vi "실습 1-1.vi"() -> ()   [LabVIEW 2014]
panel:
  out "웨이브폼 차트":dbl(graph)
  in  "정지":bool
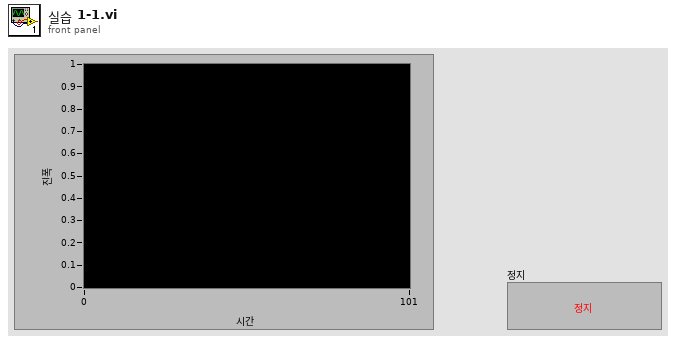
[diagram p1: front panel]
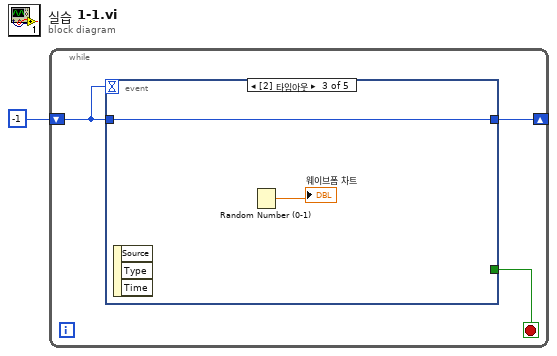
[diagram p0: block diagram]
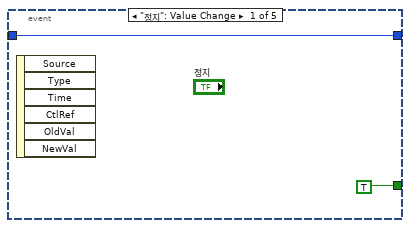
[diagram p2: hidden frame]
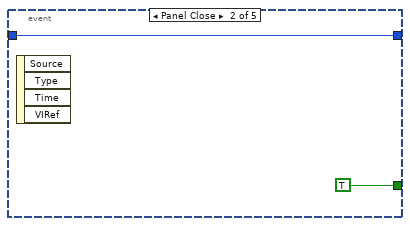
[diagram p3: hidden frame]
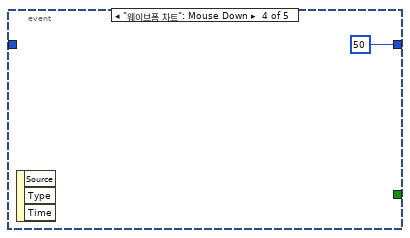
[diagram p4: hidden frame]
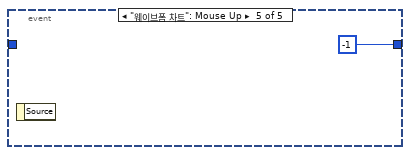
[diagram p5: hidden frame]
diagram:
  n1 = while {
    shift-right: [w3] -> _
    shift-left: -1 -> [w2]
    stop <- w4 stop-if-true
    n2 = event shown="[2] 타임아웃" {
      selector: _ -> [_ _ _ _ _]
      dyn-events: _ -> [_ _ _ _ _]
      timeout: w2 -> [_ _ _ _ _]
      tunnel: [TRUE TRUE _ _ _] -> w4
      tunnel: w2 -> [w6 w8 w10 _ _]
      tunnel: [w6 w8 w10 50 -1] -> w3
      event "정지": Value Change {
        n3 = event-data() -> ()  [unwired: 1 in, 6 out]
      }
      event Panel Close {
        n4 = event-data() -> ()  [unwired: 1 in, 4 out]
      }
      event Timeout {
        n5 = event-data() -> ()  [unwired: 1 in, 3 out]
        n6 = Random Number (0-1)() -> (number: 0 to 1=→"웨이브폼 차트":dbl)
      }
      event "웨이브폼 차트": Mouse Down {
        n7 = event-data() -> ()  [unwired: 1 in, 3 out]
      }
      event "웨이브폼 차트": Mouse Up {
        n8 = event-data() -> ()  [unwired: 1 in, 1 out]
      }
    }
  }
